vi "Begin.vi"(8 "error in":errorcluster) -> (0 "error out":errorcluster)   [LabVIEW 2018]
doc: "Called before other user functions, this VI is expected to open initial I/O refnums, load in file data, and do all program initialization. Notice that the <B>error out</B> terminal is simply used for data flow. Wiring it to other structures or subVIs ensures that this VI runs first."
uses:
  <vilib>/Rock Robotics/SystemInterfaces/DIO/FPGA_DIOPWMChannel.ctl
  <vilib>/Rock Robotics/WPI/DriverStation/WPI_DriverStationRobotMode2.ctl
  <vilib>/Rock Robotics/WPI/Joystick/WPI_JoystickDeviceEnum.ctl
  <vilib>/Rock Robotics/WPI/Solenoid/WPI_SolenoidChannel.ctl
  <vilib>/Rock Robotics/SystemInterfaces/DIO/FPGA_DIOChannel.ctl
  <vilib>/Rock Robotics/WPI/SafetyOutput/WPI_SafetyOutputConfigMenu.ctl
  Robot Global Data.vi
  <vilib>/Rock Robotics/Network Tables/NT Write String Array.vi
  <vilib>/Rock Robotics/WPI/RobotDrive/WPI_RobotDriveOpen4MotorWithTalonSRX.vi
  <vilib>/Rock Robotics/WPI/Solenoid/WPI_SolenoidOpenSingle.vi
  <vilib>/Rock Robotics/WPI/Switch/WPI_SwitchOpenLimit.vi
  <vilib>/Rock Robotics/WPI/MotorControl/WPI_MotorControlOpen TalonSRX.vi
  Global 1.vi
  <vilib>/Rock Robotics/WPI/Counter/WPI_CounterDigitalInputToDigitalSource.vi
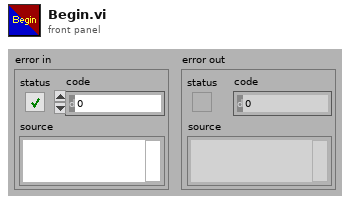
[diagram p1: front panel]
types:
  T1 = typedef "FPGA_DIOChannel.ctl" = enum8{"DIO 0", "DIO 1", "DIO 2", "DIO 3", "DIO 4", "DIO 5", "DIO 6", "DIO 7", "DIO 8", "DIO 9", "DIO MXP 0", "DIO MXP 1", "DIO MXP 2", "DIO MXP 3", "DIO MXP 4", "DIO MXP 5", "DIO MXP 6", "DIO MXP 7", "DIO MXP 8", "DIO MXP 9", "DIO MXP 10", "DIO MXP 11", "DIO MXP 12", "DIO MXP 13", "DIO MXP 14", "DIO MXP 15", "SPI Port CS1", "SPI Port CS2", "SPI Port CS3", "SPI Port MISO", "SPI Port MOSI", "Invalid"}
  T2 = typedef "WPI_SafetyOutputConfigMenu.ctl" = enum16{"Enable", "Disable"}
  T3 = typedef "FPGA_DIOPWMChannel.ctl" = enum8{"PWM 0", "PWM 1", "PWM 2", "PWM 3", "PWM 4", "PWM 5", "PWM 6", "PWM 7", "PWM 8", "PWM 9", "PWM MXP 0", "PWM MXP 1", "PWM MXP 2", "PWM MXP 3", "PWM MXP 4", "PWM MXP 5", "PWM MXP 6", "PWM MXP 7", "PWM MXP 8", "PWM MXP 9", "Invalid"}
  T4 = enum16{"FollowerType_PercentOutput", "FollowerType_AuxOutput1"}
  T5 = typedef "WPI_JoystickDeviceEnum.ctl" = enum16{"USB 0", "USB 1", "USB 2", "USB 3", "USB 4", "USB 5"}
  T6 = typedef "WPI_SolenoidChannel.ctl" = enum8{"Solenoid 0", "Solenoid 1", "Solenoid 2", "Solenoid 3", "Solenoid 4", "Solenoid 5", "Solenoid 6", "Solenoid 7", "Invalid"}
  T7 = typedef "WPI_DriverStationRobotMode2.ctl" = enum16{"Autonomous Disabled", "Autonomous Enabled", "Teleop Disabled", "Teleop Enabled", "Disconnected", "Finish", "Test Disabled", "Test Enabled", "Emergency Stopped"}
  T8 = typedef "WPI_MotorControlDeviceRef.ctl" = cluster{"DeviceStatus":errorcluster, "Type":T9, "PWM":cluster{"PWM Channel":T3, "DeadBand":T10}, "CAN":cluster{"Device Number":u8, "SetOutput VI Ref":variant, "GetOutput VI Ref":variant, "Enable VI Ref":variant, "Disable VI Ref":variant, "Data":variant}, "Invert":bool, "DIO PWM":cluster{"PWM \"Enable\" Channel":T3, "DIOChannel":T1, "PWM Rate":dbl}}
  T9 = typedef "WPI_MotorControlType.ctl" = enum16{"PWM", "CAN", "DIO PWM"}
  T10 = typedef "WPI_PWMDeadband.ctl" = cluster{"Name":string, "maxPositivePwm":i32, "minPositivePwm":i32, "centerPwm":i32, "maxNegativePwm":i32, "minNegativePwm":i32, "angularRange":u16}
  T11 = typedef "WPI_RobotDriveDevRef.ctl" = cluster{"DevStatus":errorcluster, "Motors[]":T8[], "Square Inputs":bool, "Max Output":dbl}
  T12 = typedef "WPI_JoystickDevRef.ctl" = cluster{"Device":T5}
  T13 = typedef "WPI_DigitalInputDevRef.ctl" = cluster{"DevStatus":errorcluster, "DIO Channel":T1}
  T14 = typedef "FPGA_CounterEncoderSourceConvertionLVSourceType.ctl" = cluster{"DevStatus":errorcluster, "AnalogTriggerMode?":bool, "DigitalMode":cluster{"DIO Channel":T15}, "AnalogTriggerMode":cluster{"AnalogTriggerIndex":T16, "OutputType":T17}}
  T15 = typedef "FPGA_DIODigitalSourceChannel.ctl" = enum8{"DIO 0", "DIO 1", "DIO 2", "DIO 3", "DIO 4", "DIO 5", "DIO 6", "DIO 7", "DIO 8", "DIO 9", "DIO MXP 0", "DIO MXP 1", "DIO MXP 2", "DIO MXP 3", "DIO MXP 4", "DIO MXP 5", "DIO MXP 6", "DIO MXP 7", "DIO MXP 8", "DIO MXP 9", "DIO MXP 10", "DIO MXP 11", "DIO MXP 12", "DIO MXP 13", "DIO MXP 14", "DIO MXP 15", "SPI Port CS1", "SPI Port CS2", "SPI Port CS3", "SPI Port MISO", "SPI Port MOSI", "Disabled"}
  T16 = typedef "FPGA_AnalogTriggerIndex.ctl" = enum8{"Trig 0", "Trig 1", "Trig 2", "Trig 3", "Trig 4", "Trig 5", "Trig 6", "Trig 7", "Invalid"}
  T17 = typedef "FPGA_AnalogTriggerOutType.ctl" = enum16{"InWindow", "TriggerState", "Rising", "Falling"}
  T18 = typedef "WPI_EncoderDevRef.ctl" = cluster{"DevStatus":errorcluster, "EncoderIndex":T19, "CounterIndex":T20, "DistancePerCount":dbl, "Decoding Type":T21}
  T19 = typedef "FPGA_EncoderIdx.ctl" = enum8{"Enc 0", "Enc 1", "Enc 2", "Enc 3", "Enc 4", "Enc 5", "Enc 6", "Enc 7", "Invalid"}
  T20 = typedef "FPGA_CounterCtrSystemIndex.ctl" = enum8{"Ctr 0", "Ctr 1", "Ctr 2", "Ctr 3", "Ctr 4", "Ctr 5", "Ctr 6", "Ctr 7", "Invalid"}
  T21 = typedef "WPI_EncoderType.ctl" = enum16{"1x", "2x", "4x"}
  T22 = typedef "WPI_SolenoidDevRef.ctl" = cluster{"DevStatus":errorcluster, "Pneumatics Control Module":u8, "Forward Solenoid Channel":T6, "Reverse Solenoid Channel":T6}
  T23 = typedef "WPI_SwitchDevRef.ctl" = cluster{"DevStatus":errorcluster, "DIO Channel":T1, "CntIndex":T20, "Normally Closed":bool}
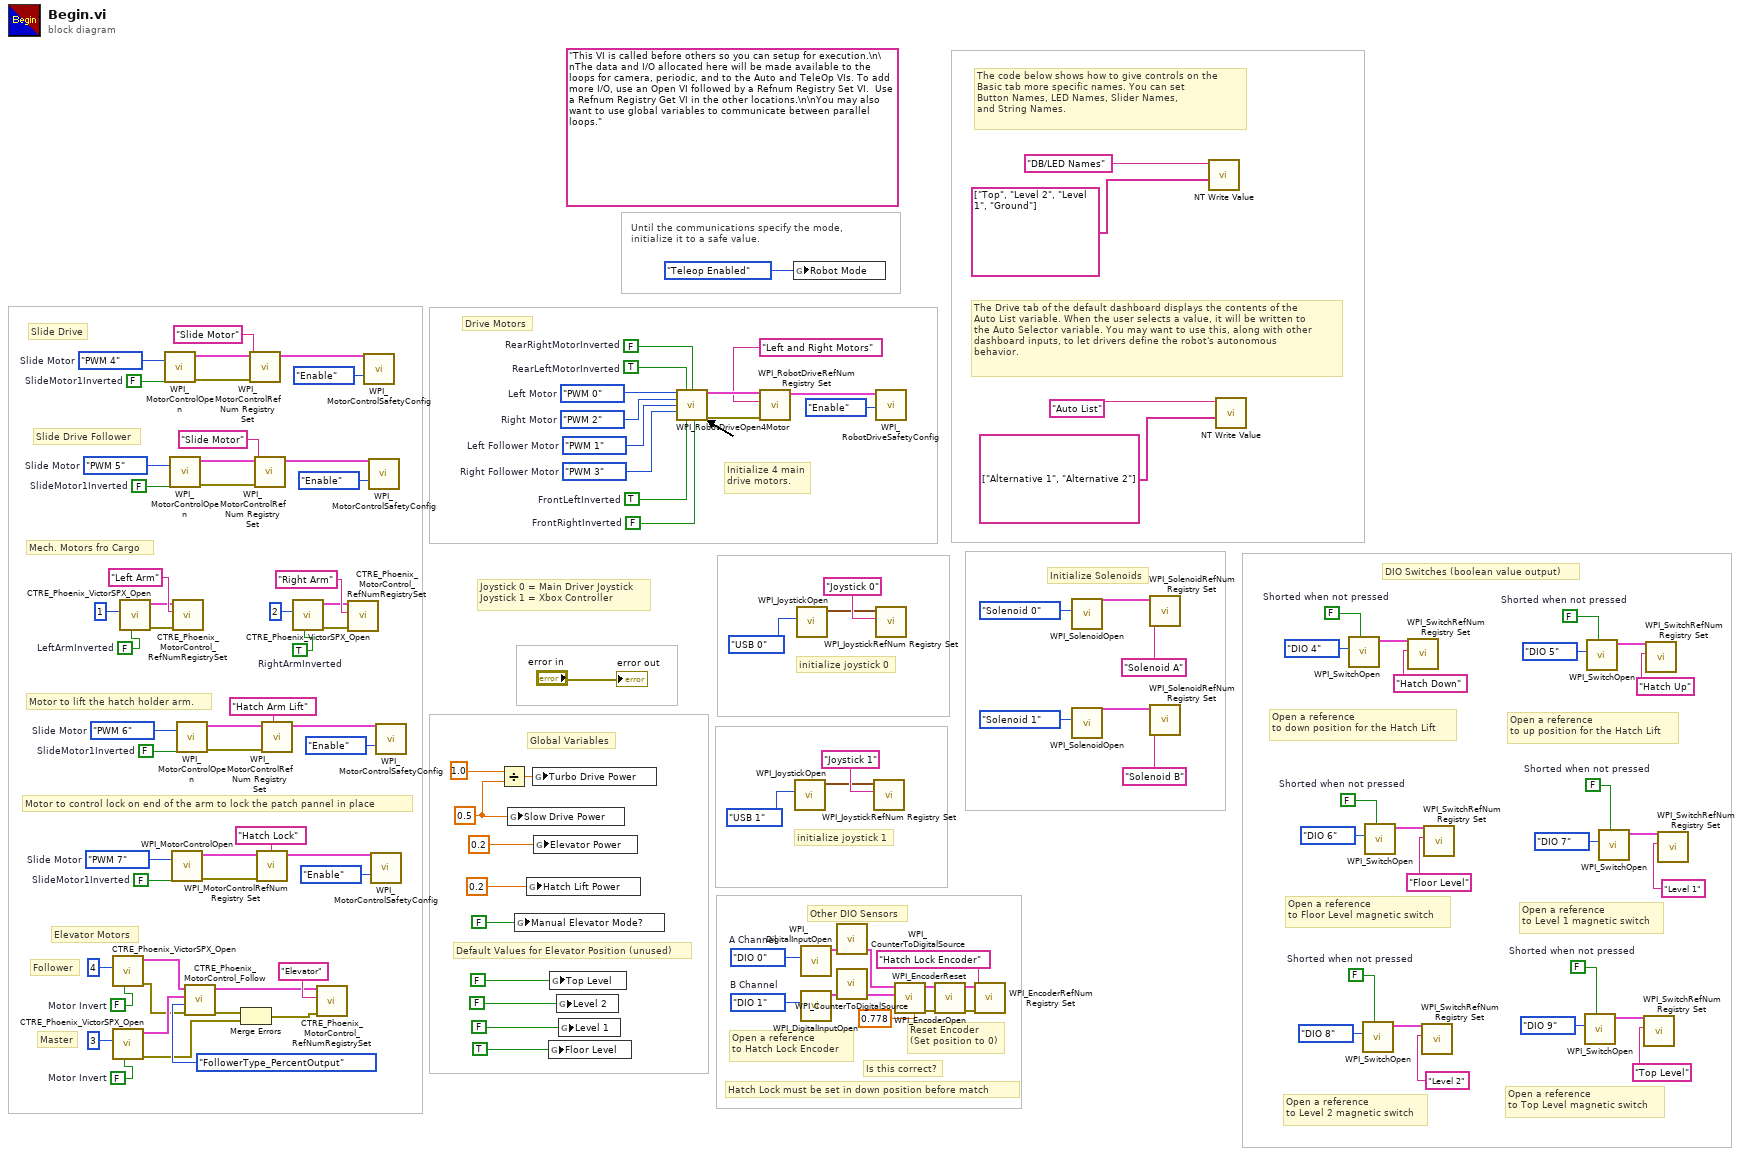
[diagram p0: block diagram]
diagram:
  w12 = FPGA_DIOChannel."DIO 1"  # B Channel
  w11 = FPGA_DIOChannel."DIO 0"  # A Channel
  w14 = FALSE  # Shorted when not pressed
  w18 = FALSE  # Shorted when not pressed
  w28 = FALSE  # SlideMotor1Inverted
  w33 = FPGA_DIOPWMChannel."PWM 7"  # Slide Motor
  w35 = FALSE  # SlideMotor1Inverted
  w40 = FPGA_DIOPWMChannel."PWM 6"  # Slide Motor
  w45 = FALSE  # Motor Invert
  w57 = FALSE  # SlideMotor1Inverted
  w63 = FPGA_DIOPWMChannel."PWM 5"  # Slide Motor
  w56 = TRUE  # RightArmInverted
  w52 = FALSE  # LeftArmInverted
  w66 = 0.5
  w47 = FALSE  # Motor Invert
  w76 = FALSE  # Shorted when not pressed
  w79 = FALSE  # SlideMotor1Inverted
  w85 = FPGA_DIOPWMChannel."PWM 4"  # Slide Motor
  w88 = FALSE  # Shorted when not pressed
  w89 = FALSE  # Shorted when not pressed
  w90 = FALSE  # Shorted when not pressed
  w107 = TRUE  # FrontLeftInverted
  w108 = FALSE  # FrontRightInverted
  w109 = FPGA_DIOPWMChannel."PWM 3"  # Right Follower Motor
  w110 = FPGA_DIOPWMChannel."PWM 1"  # Left Follower Motor
  (unwired) "This VI is called before others so you can setup for execution.\n\nThe data and I/O allocated here will be made available to the loops for camera, periodic, and to the Auto and TeleOp VIs. To add more I/O, use an Open VI followed by a Refnum Registry Set VI.  Use a Refnum Registry Get VI in the other locations.\n\nYou may also want to use global variables to communicate between parallel loops."
  w122 = FPGA_DIOPWMChannel."PWM 2"  # Right Motor
  w123 = FPGA_DIOPWMChannel."PWM 0"  # Left Motor
  w127 = TRUE  # RearLeftMotorInverted
  w128 = FALSE  # RearRightMotorInverted
  # "Hatch Lock must be set in down position before match"
  # "Is this correct?"
  # "Reset Encoder\n(Set position to 0)"
  # "Open a reference\nto Hatch Lock Encoder"
  # "Other DIO Sensors"
  # "DIO Switches (boolean value output)"
  # "Open a reference\nto up position for the Hatch Lift"
  # "Open a reference\nto down position for the Hatch Lift"
  # "Default Values for Elevator Position (unused)"
  # "Elevator Motors"
  # "Motor to control lock on end of the arm to lock the patch pannel in place"
  # "Motor to lift the hatch holder arm."
  # "Global Variables"
  # "Follower"
  # "Master"
  # "Slide Drive Follower"
  # "Slide Drive"
  # "Open a reference\nto Top Level magnetic switch"
  # "Drive Motors"
  # "Mech. Motors fro Cargo"
  # "Open a reference\nto Level 2 magnetic switch"
  # "Open a reference\nto Level 1 magnetic switch"
  # "Open a reference\nto Floor Level magnetic switch"
  # "Initialize Solenoids"
  # "Initialize 4 main\ndrive motors."
  # "Joystick 0 = Main Driver Joystick\nJoystick 1 = Xbox Controller"
  # "initialize joystick 1"
  # "The Drive tab of the default dashboard displays the contents of the\nAuto List variable. When the user selects a value, it will be written to\nthe Auto Selector variable. You may want to use this, along with other\ndashboard inputs, to let drivers define the robot's autonomous\nbehavior."
  # "The code below shows how to give controls on the\nBasic tab more specific names. You can set\nButton Names, LED Names, Slider Names,\nand String Names."
  # "initialize joystick 0"
  # "Until the communications specify the mode,\ninitialize it to a safe value."
  n1 = call "CTRE_Phoenix_VictorSPX_Open.vi"("Invert"=w47, "Device Number"=u8 4) -> ("error out"=w24:errorcluster, "CAN Talon SRX Ref"=w43:T8)  [unwired: 8 in]
  n2 = call "CTRE_Phoenix_VictorSPX_Open.vi"("Invert"=w45, "Device Number"=u8 3) -> ("error out"=w23:errorcluster, "CAN Talon SRX Ref"=w44:T8)  [unwired: 8 in]
  n3 = call "CTRE_Phoenix_VictorSPX_Open.vi"("Invert"=w52, "Device Number"=u8 1) -> ("error out"=w49:errorcluster, "CAN Talon SRX Ref"=w50:T8)  [unwired: 8 in]
  n4 = call-poly <vilib>:"WPI_MotorControlOpen.vi"("Invert"=w79, "PWM Channel"=w85) -> ("error out"=w83:errorcluster, "MotorControlDeviceRef"=w84:T8)  [unwired: 8 in]
  n5 = call-poly <vilib>:"WPI_MotorControlOpen.vi"("Invert"=w57, "PWM Channel"=w63) -> ("error out"=w61:errorcluster, "MotorControlDeviceRef"=w62:T8)  [unwired: 8 in]
  n6 = call-poly <vilib>:"WPI_MotorControlOpen.vi"("Invert"=w28, "PWM Channel"=w33) -> ("error out"=w31:errorcluster, "MotorControlDeviceRef"=w32:T8)  [unwired: 8 in]
  n7 = call "CTRE_Phoenix_MotorControl_RefNumRegistrySet.vi"("error in (no error)"=w49, "refnum name"="Left Arm", "PhoenixMotorControlDevRef"=w50) -> ()  [unwired: 7 in, 2 out]
  n8 = call-poly <vilib>:"WPI_MotorControlOpen.vi"("Invert"=w35, "PWM Channel"=w40) -> ("error out"=w38:errorcluster, "MotorControlDeviceRef"=w39:T8)  [unwired: 8 in]
  n9 = call "CTRE_Phoenix_MotorControl_Follow.vi"("error in (no error)"=w24, "FollowerType"=T4."FollowerType_PercentOutput", "Master Controller to Follow"=w44, "PhoenixMotorControlDevRef"=w43) -> ("error out"=w25:errorcluster, "PhoenixMotorControlDevRef"=w42:T8)  [unwired: 6 in]
  n10 = Merge Errors(w25, w23) -> (w26:errorcluster)
  n11 = call <vilib>:"WPI_MotorControlRefNum Registry Set.vi"("error in (no error)"=w83, "refnum name"="Slide Motor", "MotorControlDevRef"=w84) -> ("MotorControlDevRef"=w81:T8)  [unwired: 7 in, 1 out]
  n12 = call <vilib>:"WPI_MotorControlRefNum Registry Set.vi"("error in (no error)"=w61, "refnum name"="Slide Motor", "MotorControlDevRef"=w62) -> ("MotorControlDevRef"=w59:T8)  [unwired: 7 in, 1 out]
  n13 = call <vilib>:"WPI_MotorControlRefNum Registry Set.vi"("error in (no error)"=w31, "refnum name"="Hatch Lock", "MotorControlDevRef"=w32) -> ("MotorControlDevRef"=w30:T8)  [unwired: 7 in, 1 out]
  n14 = call <vilib>:"WPI_MotorControlRefNum Registry Set.vi"("error in (no error)"=w38, "refnum name"="Hatch Arm Lift", "MotorControlDevRef"=w39) -> ("MotorControlDevRef"=w37:T8)  [unwired: 7 in, 1 out]
  n15 = call "CTRE_Phoenix_VictorSPX_Open.vi"("Invert"=w56, "Device Number"=u8 2) -> ("error out"=w53:errorcluster, "CAN Talon SRX Ref"=w54:T8)  [unwired: 8 in]
  n16 = call "CTRE_Phoenix_MotorControl_RefNumRegistrySet.vi"("error in (no error)"=w26, "refnum name"="Elevator", "PhoenixMotorControlDevRef"=w42) -> ()  [unwired: 7 in, 2 out]
  n17 = call "CTRE_Phoenix_MotorControl_RefNumRegistrySet.vi"("error in (no error)"=w53, "refnum name"="Right Arm", "PhoenixMotorControlDevRef"=w54) -> ()  [unwired: 7 in, 2 out]
  n18 = call <vilib>:"WPI_MotorControlSafetyConfig.vi"("mode"=WPI_SafetyOutputConfigMenu."Enable", "MotorControlDevRef"=w81) -> ()  [unwired: 8 in, 2 out]
  n19 = call <vilib>:"WPI_MotorControlSafetyConfig.vi"("mode"=WPI_SafetyOutputConfigMenu."Enable", "MotorControlDevRef"=w59) -> ()  [unwired: 8 in, 2 out]
  n20 = call <vilib>:"WPI_MotorControlSafetyConfig.vi"("mode"=WPI_SafetyOutputConfigMenu."Enable", "MotorControlDevRef"=w30) -> ()  [unwired: 8 in, 2 out]
  n21 = call <vilib>:"WPI_MotorControlSafetyConfig.vi"("mode"=WPI_SafetyOutputConfigMenu."Enable", "MotorControlDevRef"=w37) -> ()  [unwired: 8 in, 2 out]
  n22 = Divide(x=1.0, y=w66) -> (x/y=w72:dbl)
  n23 = global write "Global 1.vi" "Slow Drive Power"(w66) -> ()
  n24 = global write "Global 1.vi" "Manual Elevator Mode?"(FALSE) -> ()
  n25 = global write "Global 1.vi" "Hatch Lift Power"(0.2) -> ()
  n26 = global write "Global 1.vi" "Turbo Drive Power"(w72) -> ()
  n27 = global write "Global 1.vi" "Elevator Power"(0.2) -> ()
  n28 = global write "Global 1.vi" "Floor Level"(TRUE) -> ()
  n29 = global write "Global 1.vi" "Top Level"(FALSE) -> ()
  n30 = global write "Global 1.vi" "Level 2"(FALSE) -> ()
  n31 = global write "Global 1.vi" "Level 1"(FALSE) -> ()
  n32 = call-poly <vilib>:"WPI_RobotDriveOpen4Motor.vi"("Rear Left Motor"=w123, "Rear Left Motor Inverted"=w127, "Rear Right Motor Inverted"=w128, "Rear Right Motor"=w122, "Front Left Motor"=w110, "Front Right Motor"=w109, "Front Left Motor Inverted"=w107, "Front Right Motor Inverted"=w108) -> ("RobotDriveDevRef"=w126:T11, "error out"=w124:errorcluster)  [unwired: 6 in]
  n33 = call <vilib>:"WPI_RobotDriveRefNum Registry Set.vi"("error in (no error)"=w124, "refnum name"="Left and Right Motors", "RobotDriveDevRef"=w126) -> ("RobotDriveDevRef"=w121:T11)  [unwired: 1 in, 7 out]
  n34 = global write "Robot Global Data.vi" "Robot Mode"(WPI_DriverStationRobotMode2."Teleop Enabled" ("Robot Mode")) -> ()
  n35 = call <vilib>:"WPI_JoystickOpen.vi"("JoystickDevice"=WPI_JoystickDeviceEnum."USB 1") -> ("JoystickDevRef"=w99:T12)  [unwired: 10 in]
  n36 = call <vilib>:"WPI_JoystickOpen.vi"("JoystickDevice"=WPI_JoystickDeviceEnum."USB 0") -> ("JoystickDevRef"=w117:T12)  [unwired: 10 in]
  n37 = call <vilib>:"WPI_DigitalInputOpen.vi"("DIO Channel"=w11) -> ("DigitalInputDevRef"=w8:T13)  [unwired: 1 in, 9 out]
  n38 = call <vilib>:"WPI_DigitalInputOpen.vi"("DIO Channel"=w12) -> ("DigitalInputDevRef"=w9:T13)  [unwired: 1 in, 9 out]
  n39 = call-poly <vilib>:"WPI_CounterToDigitalSource.vi"("DigitalInputDevRef"=w8) -> ("Digital Source"=w7:T14)  [unwired: 6 out]
  n40 = call-poly <vilib>:"WPI_CounterToDigitalSource.vi"("DigitalInputDevRef"=w9) -> ("Digital Source"=w10:T14)  [unwired: 6 out]
  n41 = call <vilib>:"WPI_JoystickRefNum Registry Set.vi"("refnum name"="Joystick 1", "JoystickDevRef"=w99) -> ()  [unwired: 8 in, 2 out]
  n42 = call <vilib>:"WPI_RobotDriveSafetyConfig.vi"("mode"=WPI_SafetyOutputConfigMenu."Enable", "RobotDriveDevRef"=w121) -> ()  [unwired: 8 in, 2 out]
  n43 = call <vilib>:"WPI_JoystickRefNum Registry Set.vi"("refnum name"="Joystick 0", "JoystickDevRef"=w117) -> ()  [unwired: 8 in, 2 out]
  n44 = call <vilib>:"WPI_EncoderOpen.vi"("DistancePerCount"=0.778, "BSource"=w10, "ASource"=w7) -> ("error out"=w4:errorcluster, "EncoderDevRef"=w3:T18)  [unwired: 5 in, 2 out]
  n45 = call <vilib>:"WPI_EncoderReset.vi"("error in (no error)"=w4, "EncoderDevRef"=w3) -> ("error out"=w1:errorcluster, "EncoderDevRef"=w2:T18)  [unwired: 8 in]
  n46 = call <vilib>:"WPI_EncoderRefNum Registry Set.vi"("error in (no error)"=w1, "refnum name"="Hatch Lock Encoder", "EncoderDevRef"=w2) -> ()  [unwired: 7 in, 2 out]
  n47 = call-poly <vilib>:"WPI_SolenoidOpen.vi"("Solenoid Channel"=WPI_SolenoidChannel."Solenoid 0") -> ("SolenoidDevRef"=w105:T22)  [unwired: 9 in, 1 out]
  n48 = call-poly <vilib>:"WPI_SolenoidOpen.vi"("Solenoid Channel"=WPI_SolenoidChannel."Solenoid 1") -> ("SolenoidDevRef"=w102:T22)  [unwired: 9 in, 1 out]
  n49 = call <vilib>:"WPI_SolenoidRefNum Registry Set.vi"("refnum name"="Solenoid A", "SolenoidDevRef"=w105) -> ()  [unwired: 8 in, 2 out]
  n50 = call <vilib>:"WPI_SolenoidRefNum Registry Set.vi"("refnum name"="Solenoid B", "SolenoidDevRef"=w102) -> ()  [unwired: 8 in, 2 out]
  n51 = call-poly <vilib>:"NT Write Value.vi"("String Array"=string[] ["Top", "Level 2", "Level 1", "Ground"], "Name"="DB/LED Names") -> ()  [unwired: 9 in, 1 out]
  n52 = call-poly <vilib>:"NT Write Value.vi"("String Array"=string[] ["Alternative 1", "Alternative 2"], "Name"="Auto List") -> ()  [unwired: 9 in, 1 out]
  n53 = call-poly <vilib>:"WPI_SwitchOpen.vi"("Normally Closed"=w18, "DIO Channel"=FPGA_DIOChannel."DIO 4") -> ("SwitchDevRef"=w21:T23)  [unwired: 8 in, 1 out]
  n54 = call-poly <vilib>:"WPI_SwitchOpen.vi"("Normally Closed"=w88, "DIO Channel"=FPGA_DIOChannel."DIO 8") -> ("SwitchDevRef"=w93:T23)  [unwired: 8 in, 1 out]
  n55 = call-poly <vilib>:"WPI_SwitchOpen.vi"("Normally Closed"=w90, "DIO Channel"=FPGA_DIOChannel."DIO 6") -> ("SwitchDevRef"=w97:T23)  [unwired: 8 in, 1 out]
  n56 = call <vilib>:"WPI_SwitchRefNum Registry Set.vi"("refnum name"="Hatch Down", "SwitchDevRef"=w21) -> ()  [unwired: 8 in, 2 out]
  n57 = call <vilib>:"WPI_SwitchRefNum Registry Set.vi"("refnum name"="Level 2", "SwitchDevRef"=w93) -> ()  [unwired: 8 in, 2 out]
  n58 = call <vilib>:"WPI_SwitchRefNum Registry Set.vi"("refnum name"="Floor Level", "SwitchDevRef"=w97) -> ()  [unwired: 8 in, 2 out]
  n59 = call-poly <vilib>:"WPI_SwitchOpen.vi"("Normally Closed"=w76, "DIO Channel"=FPGA_DIOChannel."DIO 9") -> ("SwitchDevRef"=w78:T23)  [unwired: 8 in, 1 out]
  n60 = call-poly <vilib>:"WPI_SwitchOpen.vi"("Normally Closed"=w14, "DIO Channel"=FPGA_DIOChannel."DIO 5") -> ("SwitchDevRef"=w17:T23)  [unwired: 8 in, 1 out]
  n61 = call-poly <vilib>:"WPI_SwitchOpen.vi"("Normally Closed"=w89, "DIO Channel"=FPGA_DIOChannel."DIO 7") -> ("SwitchDevRef"=w95:T23)  [unwired: 8 in, 1 out]
  n62 = call <vilib>:"WPI_SwitchRefNum Registry Set.vi"("refnum name"="Top Level", "SwitchDevRef"=w78) -> ()  [unwired: 8 in, 2 out]
  n63 = call <vilib>:"WPI_SwitchRefNum Registry Set.vi"("refnum name"="Hatch Up", "SwitchDevRef"=w17) -> ()  [unwired: 8 in, 2 out]
  n64 = call <vilib>:"WPI_SwitchRefNum Registry Set.vi"("refnum name"="Level 1", "SwitchDevRef"=w95) -> ()  [unwired: 8 in, 2 out]
  "error out" <- "error in"
